vi "Close TDMS File.vi"(8 "error in (no error)":errorcluster, 11 "TDMS-Actor in":refnum<class "TDMS-Actor.lvclass">) -> (0 "error out":errorcluster, 3 "TDMS-Actor out":refnum<class "TDMS-Actor.lvclass">)   [LabVIEW 2014, in "BNT_TDMS.lvlib" / "TDMS-Actor.lvclass"]
doc: "Close TDMS file."
uses:
  TDMS-Actor.lvclass
  TDMS-Actor.lvclass/TDMS-Actor.ctl
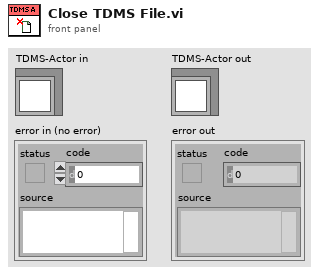
[diagram p1: front panel]
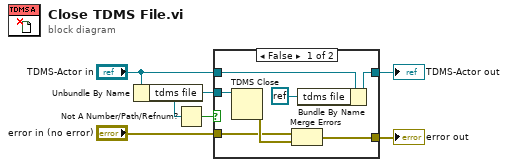
[diagram p0: block diagram]
diagram:
  n1 = Unbundle By Name("TDMS-Actor in") -> ("tdms file"=w2:refnum<k34>)
  n2 = Not A Number/Path/Refnum?(number/path/refnum=w2) -> (NaN/Path/Refnum?=w1:bool)
  n3 = case shown="False" w1 {
    tunnel: w2 -> [w13 _]
    tunnel: "error in (no error)" -> [w7 w15]
    tunnel: [w8 w15] -> w5
    tunnel: "TDMS-Actor in" -> [w11 w14]
    tunnel: [w9 w14] -> w3
    frame False {
      n4 = TDMS Close(11:w13) -> (0:w12:errorcluster)  [unwired: 1 in, 1 out]
      n5 = Merge Errors(w7, w12) -> (w8:errorcluster)
      n6 = Bundle By Name(cluster=w11, "tdms file"=refnum<k0> refnum) -> (w9:refnum<class "TDMS-Actor.lvclass">)
    }
    frame True {
    }
  }
  "error out" <- w5
  "TDMS-Actor out" <- w3
